vi "Get Gyro.vi"(11 "Gyro ID (1 or 2)":i32) -> (1 "Rate":dbl, 2 "Angle":dbl)   [LabVIEW 2015]
doc: "Gets a gyro angle/rate."
uses:
  Gyro Global.vi
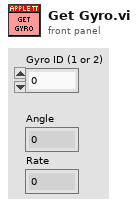
[diagram p1: front panel]
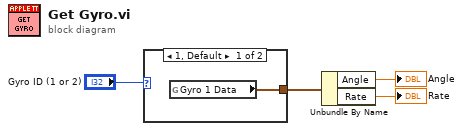
[diagram p0: block diagram]
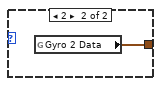
[diagram p2: hidden frame]
diagram:
  n1 = case shown="1, Default" "Gyro ID (1 or 2)" {
    tunnel: [w5 w6] -> w1
    frame 1, Default {
      n2 = global read "Gyro Global.vi" "Gyro 1 Data"() -> (w5:cluster{"Rate":dbl, "Angle":dbl, "Gain":dbl})
    }
    frame 2 {
      n3 = global read "Gyro Global.vi" "Gyro 2 Data"() -> (w6:cluster{"Rate":dbl, "Angle":dbl, "Gain":dbl})
    }
  }
  n4 = Unbundle By Name(w1) -> ("Angle"=→"Angle":dbl, "Rate"=→"Rate":dbl)
